vi "Settings2.vi"(10 "Array":dbl[](array[numeric]), 11 "Enable":bool) -> (3 "Numeric Indicator":dbl)   [LabVIEW 2011]
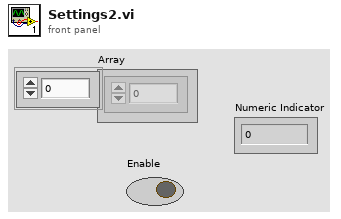
[diagram p1: front panel]
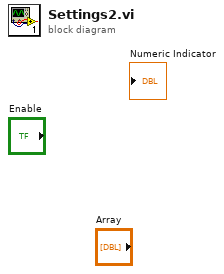
[diagram p0: block diagram]
diagram:
